vi "CheckAccTimes.vi"(8 "错误输入（无错误）":errorcluster, 11 "采样数据累积次数":u32) -> (0 "错误输出":errorcluster, 3 "返回值":i32)   [LabVIEW 2014]
uses:
  X86Dll/ZXUTConfigMgr.dll
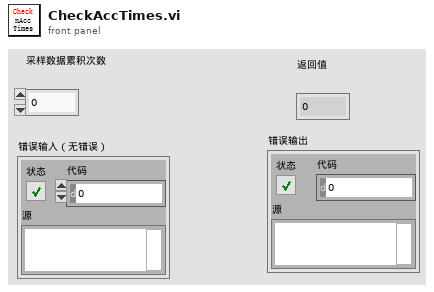
[diagram p1: front panel]
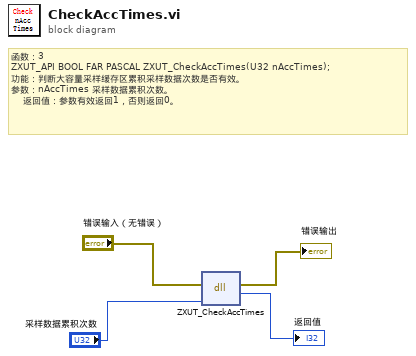
[diagram p0: block diagram]
diagram:
  # "函数：3\nZXUT_API BOOL\tFAR PASCAL ZXUT_CheckAccTimes(U32 nAccTimes);\n功能：判断大容量采样缓存区累积采样数据次数是否有效。\n参数：nAccTimes 采样数据累积次数。\n\t   返回值：参数有效返回1，否则返回0。"
  n1 = dll-call lib="D:/Software/Utrasonic on-line monitoring/X86Dll/ZXUTConfigMgr.dll" fn="ZXUT_CheckAccTimes"(error in="错误输入（无错误）", "nAccTimes"="采样数据累积次数") -> (error out=→"错误输出":errorcluster, "返回值"=→"返回值":i32)  [unwired: 3 in, 1 out]
